vi "Add Menu Items.vi"(0 "Menu in":refnum<k9>, 2 "Menu Items":T1(array[cluster]), 5 "index":i32, 9 "menu tag":string, 11 "error in (no error)":errorcluster) -> (4 "Menu out":refnum<k9>, 15 "error out":errorcluster)   [LabVIEW 2015, in "KMultilevel Ring.xctl"]
uses:
  KMultilevel Ring.xctl
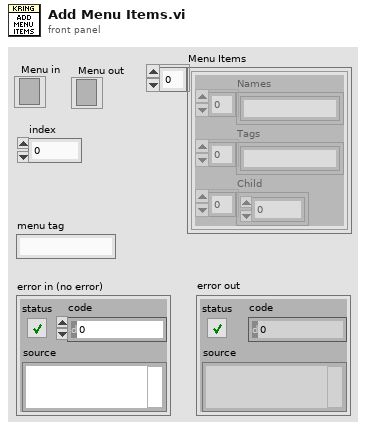
[diagram p1: front panel]
types:
  T1 = cluster{"Names":string[], "Tags":string[], "Child":i32[]}[]
  T2 = cluster{"Names":string[], "Tags":string[], "Child":i32[]}
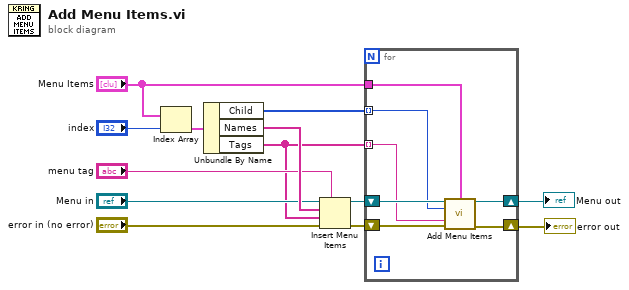
[diagram p0: block diagram]
diagram:
  n1 = Index Array(array="Menu Items", index="index") -> (element=w11:T2)
  n2 = Unbundle By Name(w11) -> ("Child"=w6:i32[], "Names"=w10:string[], "Tags"=w5:string[])
  n3 = Insert Menu Items(5:"menu tag", 6:"error in (no error)", 7:w5, 8:w10, 9:"Menu in") -> (0:w3:errorcluster, 3:w4:refnum<k9>)  [unwired: 1 in, 1 out]
  "Menu out" <- w4
  n4 = for {
    tunnel: w6 -> [w15] mode=indexing
    tunnel: w5 -> [w14] mode=indexing
    tunnel: "Menu Items" -> [w17]
    shift-right: [w16] -> w1
    shift-left: w3 -> [w18]
    shift-right: [w13] -> _
    shift-left: w4 -> [w19]
    n5 = call "Add Menu Items.vi"("Menu in"=w19, "Menu Items"=w17, "index"=w15, "menu tag"=w14, "error in (no error)"=w18) -> ("Menu out"=w13:refnum<k9>, "error out"=w16:errorcluster)  [unwired: 9 in]
  }
  "error out" <- w1
